vi "Cannon Get.vi"(0 "Motor VBus":dbl, 2 "Arm?":bool, 3 "Cannon Info":T2, 4 "Shoot":bool) -> (1 "Cannon Info 2":T2)   [LabVIEW 2013]
uses:
  <vilib>/Rock Robotics/WPI/Relay/WPI_RelayValue.ctl
  <vilib>/Rock Robotics/WPI/Solenoid/WPI_SolenoidValue.ctl
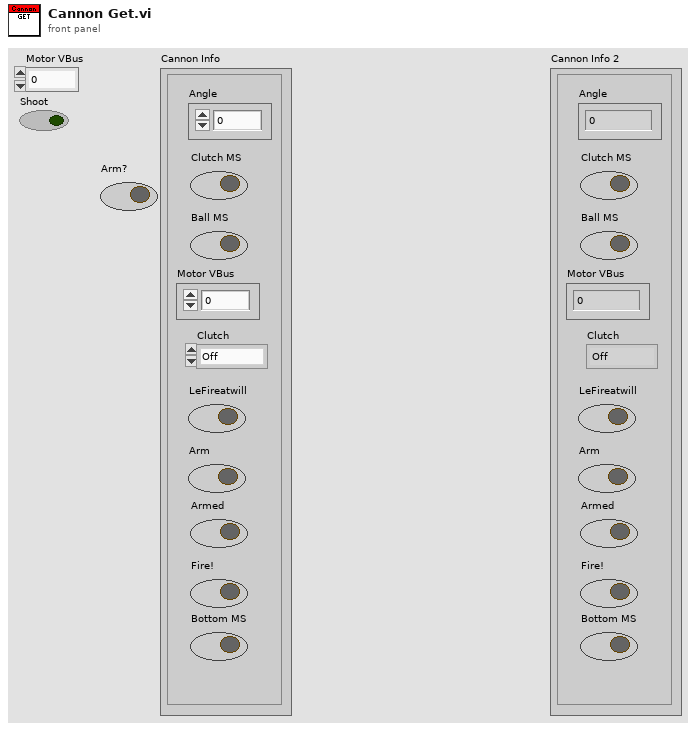
[diagram p1: front panel]
types:
  T1 = typedef "WPI_RelayValue.ctl" = enum16{"Off", "On", "Forward", "Reverse"}
  T2 = cluster{"Angle":dbl, "Clutch MS":bool, "Ball MS":bool, "Clutch ":T1, "LeFireatwill":bool, "Arm":bool, "Armed":bool, "Fire!":bool, "Bottom MS":bool, "Motor VBus":dbl}
  T3 = typedef "WPI_SolenoidValue.ctl" = enum16{"Off", "On", "Forward", "Reverse"}
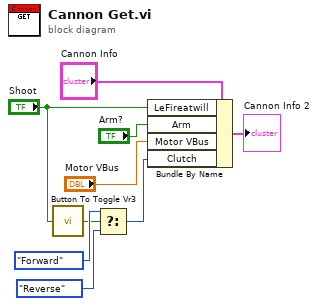
[diagram p0: block diagram]
diagram:
  n1 = call "Button To Toggle Vr3.vi"("InValue"="Shoot") -> ("Result"=w4:bool)
  n2 = Select(t=WPI_SolenoidValue."Forward" ("Value"), s=w4, f=WPI_SolenoidValue."Reverse" ("Value")) -> (s? t:f=w7:T3)
  n3 = Bundle By Name(cluster="Cannon Info", "LeFireatwill"="Shoot", "Arm"="Arm?", "Motor VBus"="Motor VBus", "Clutch"=w7) -> (→"Cannon Info 2":T2)
